vi "readTag.vi"(8 "error in (no error)":errorcluster, 11 "RaspberryPi in":refnum<class "RaspberryPi.lvclass">) -> (0 "error out":errorcluster, 3 "RaspberryPi out":refnum<class "RaspberryPi.lvclass">)   [LabVIEW 2020, in "RaspberryPi.lvclass"]
uses:
  RaspberryPi.lvclass
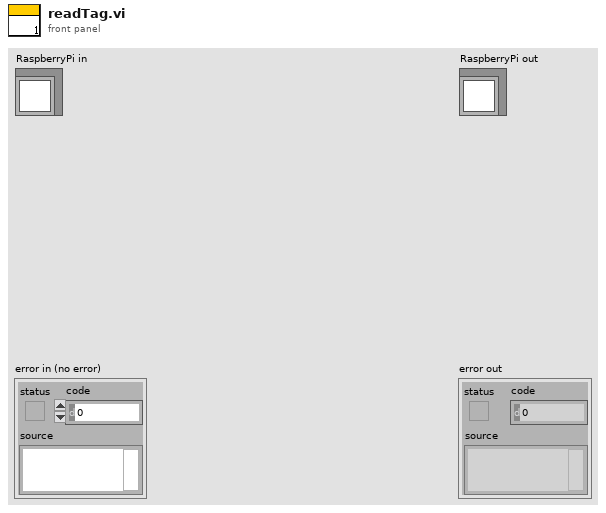
[diagram p1: front panel]
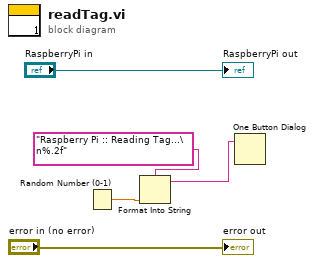
[diagram p0: block diagram]
diagram:
  n1 = Random Number (0-1)() -> (number: 0 to 1=w2:dbl)
  n2 = Format Into String(format string="Raspberry Pi :: Reading Tag...\n%.2f" ("message"), w2) -> (resulting string=w1:string)  [unwired: 2 in, 1 out]
  n3 = One Button Dialog(message=w1) -> ()  [unwired: 1 in, 1 out]
  "error out" <- "error in (no error)"
  "RaspberryPi out" <- "RaspberryPi in"
